vi "Launch menu.vi"(8 "error in (no error)":errorcluster, 9 "Menu object array.lvclass":refnum<class "Menu object array.lvclass">, 10 "Menu object names":string[](array[string])=["Select one...", "Test base", "Lockin"], 11 "Interface with menu in":refnum<class "Interface with menu.lvclass">) -> (0 "error out":errorcluster, 2 "Menu queue out":refnum<class "Message Enqueuer.lvclass">, 3 "Interface with menu out":refnum<class "Interface with menu.lvclass">)   [LabVIEW 2015, in "Interface with menu.lvclass"]
uses:
  Interface with menu.lvclass
  Menu object array/Menu object array.lvclass
  <vilib>/ActorFramework/Message Enqueuer/Message Enqueuer.lvclass
  Interface with menu.lvclass/Interface with menu.ctl
  Menu object array Messages/Write menu object names Msg/Write menu object names Msg.lvclass/Write menu object names Msg.ctl
  <vilib>/ActorFramework/Message Enqueuer/Message Enqueuer.lvclass/Message Enqueuer.ctl
  Mag Lab Measure Interface Messages/Attach to subpanel Msg/Attach to subpanel Msg.lvclass/Attach to subpanel Msg.ctl
  <vilib>/ActorFramework/Message Enqueuer/Enqueue.vi
  <vilib>/ActorFramework/Message Priority Queue/Priority Enqueue.vi
  Menu object array Messages/Write menu object names Msg/Write menu object names Msg.lvclass
  Mag Lab Measure Interface Messages/Attach to subpanel Msg/Attach to subpanel Msg.lvclass
  <vilib>/ActorFramework/Actor/Actor.lvclass
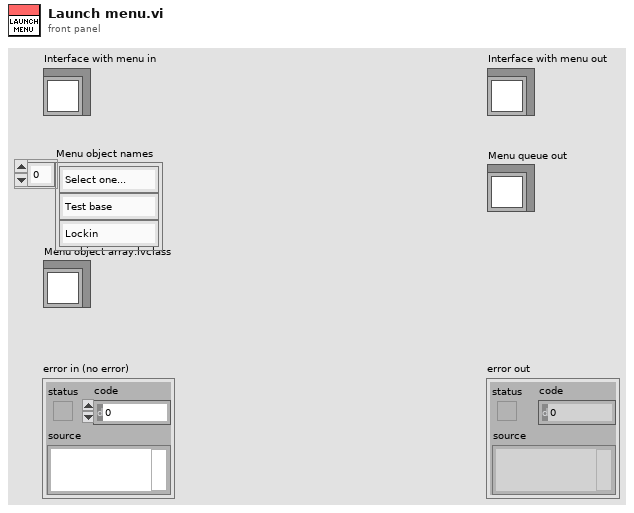
[diagram p1: front panel]
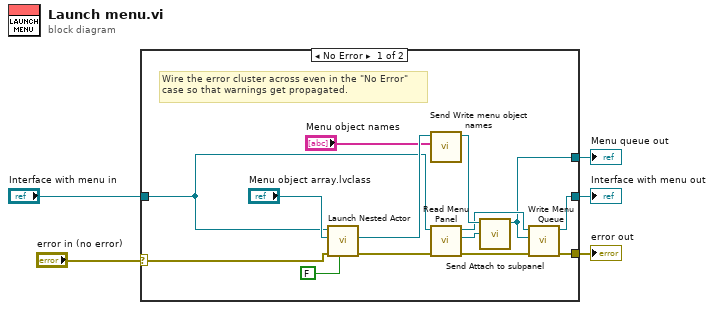
[diagram p0: block diagram]
diagram:
  n1 = case shown="No Error" "error in (no error)" {
    selector: "error in (no error)" -> [w9 w21]
    tunnel: [w11 w21] -> w4
    tunnel: [w14 w20] -> w2
    tunnel: "Interface with menu in" -> [w6 w20]
    tunnel: [w8 _] -> w1
    frame No Error {
      # "Wire the error cluster across even in the \"No Error\"\ncase so that warnings get propagated."
      n2 = call <vilib>:"Launch Nested Actor.vi"("Open Actor Core front panel? (F)"=FALSE, "error in (no error)"=w9, "Nested Actor"="Menu object array.lvclass", "Caller Actor in"=w6) -> ("error out"=w13:errorcluster, "Nested Actor's Enqueuer"=w19:refnum<class "Message Enqueuer.lvclass">)  [unwired: 5 in, 1 out]
      n3 = call "Send Write menu object names.vi"("Menu object names"="Menu object names", "Message Enqueuer"=w19) -> ("Message Enqueuer out"=w18:refnum<class "Message Enqueuer.lvclass">)  [unwired: 8 in, 1 out]
      n4 = call "Read Menu  Panel.vi"("error in (no error)"=w13, "Interface with menu in"=w6) -> ("error out"=w12:errorcluster, "Menu  Panel"=w17:refnum<vi>, "Interface with menu out"=w15:refnum<class "Interface with menu.lvclass">)  [unwired: 7 in]
      n5 = call "Send Attach to subpanel.vi"("Sub Panel"=w17, "Message Enqueuer"=w18) -> ("Message Enqueuer out"=w8:refnum<class "Message Enqueuer.lvclass">)  [unwired: 8 in, 1 out]
      n6 = call "Write Menu Queue.vi"("error in (no error)"=w12, "Actor Framework.lvlib:Message Enqueuer"=w8, "Interface with menu in"=w15) -> ("error out"=w11:errorcluster, "Interface with menu out"=w14:refnum<class "Interface with menu.lvclass">)  [unwired: 7 in]
    }
    frame Error {
    }
  }
  "error out" <- w4
  "Interface with menu out" <- w2
  "Menu queue out" <- w1
